vi "RemoveInterface.vi"(6 "InterfaceMethodsToRemove":string[](array[string])=["Add.Vi", "Execute.vi"], 7 "ClassWriter.lvclass":refnum<class "ClassWriter.lvclass">, 8 "error in":errorcluster, 9 "RemoveMethods":bool=TRUE, 10 "Interface Path":path=path "C:/Projects/Interface/Sub_Interface1/Sub_Interface1.lvclass", 11 "LvClassPath/LvClassProjectItem":variant) -> (0 "error out":errorcluster={"status"=TRUE, "code"=7, "source"="Invoke Node in InterfaceLibrary.lvlib:ImplementInterface.vi\n<APPEND>\nMethod Name: <b>LabVIEW Class:Open</b>"})   [LabVIEW 2020, in "InterfaceLibrary.lvlib"]
uses:
  InterfaceLibrary.lvlib
  Provider_BaseClassInterface/ClassWriter_class/ClassWriter.lvclass
  Provider_LvNativeClass/ClassWriterNative_class/ClassWriterNative.lvclass
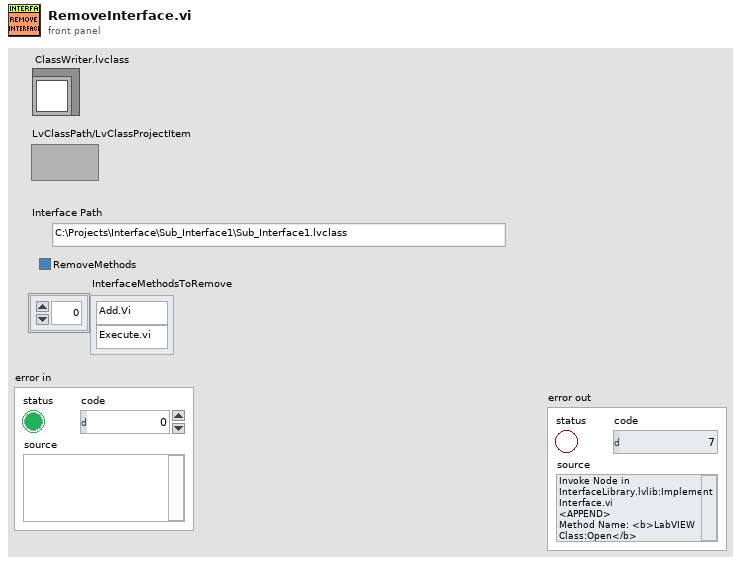
[diagram p1: front panel]
types:
  T1 = cluster{"ClassRef":refnum<vi>, "ClassRefCreated":bool, "Application":refnum<vi>, "InterfaceRef":refnum<vi>, "MethodsToImplement":path[], "MethodsDescription":string[], "MethodsScope":enum32{"invalid scope", "public", "private", "protected", "community"}[]}
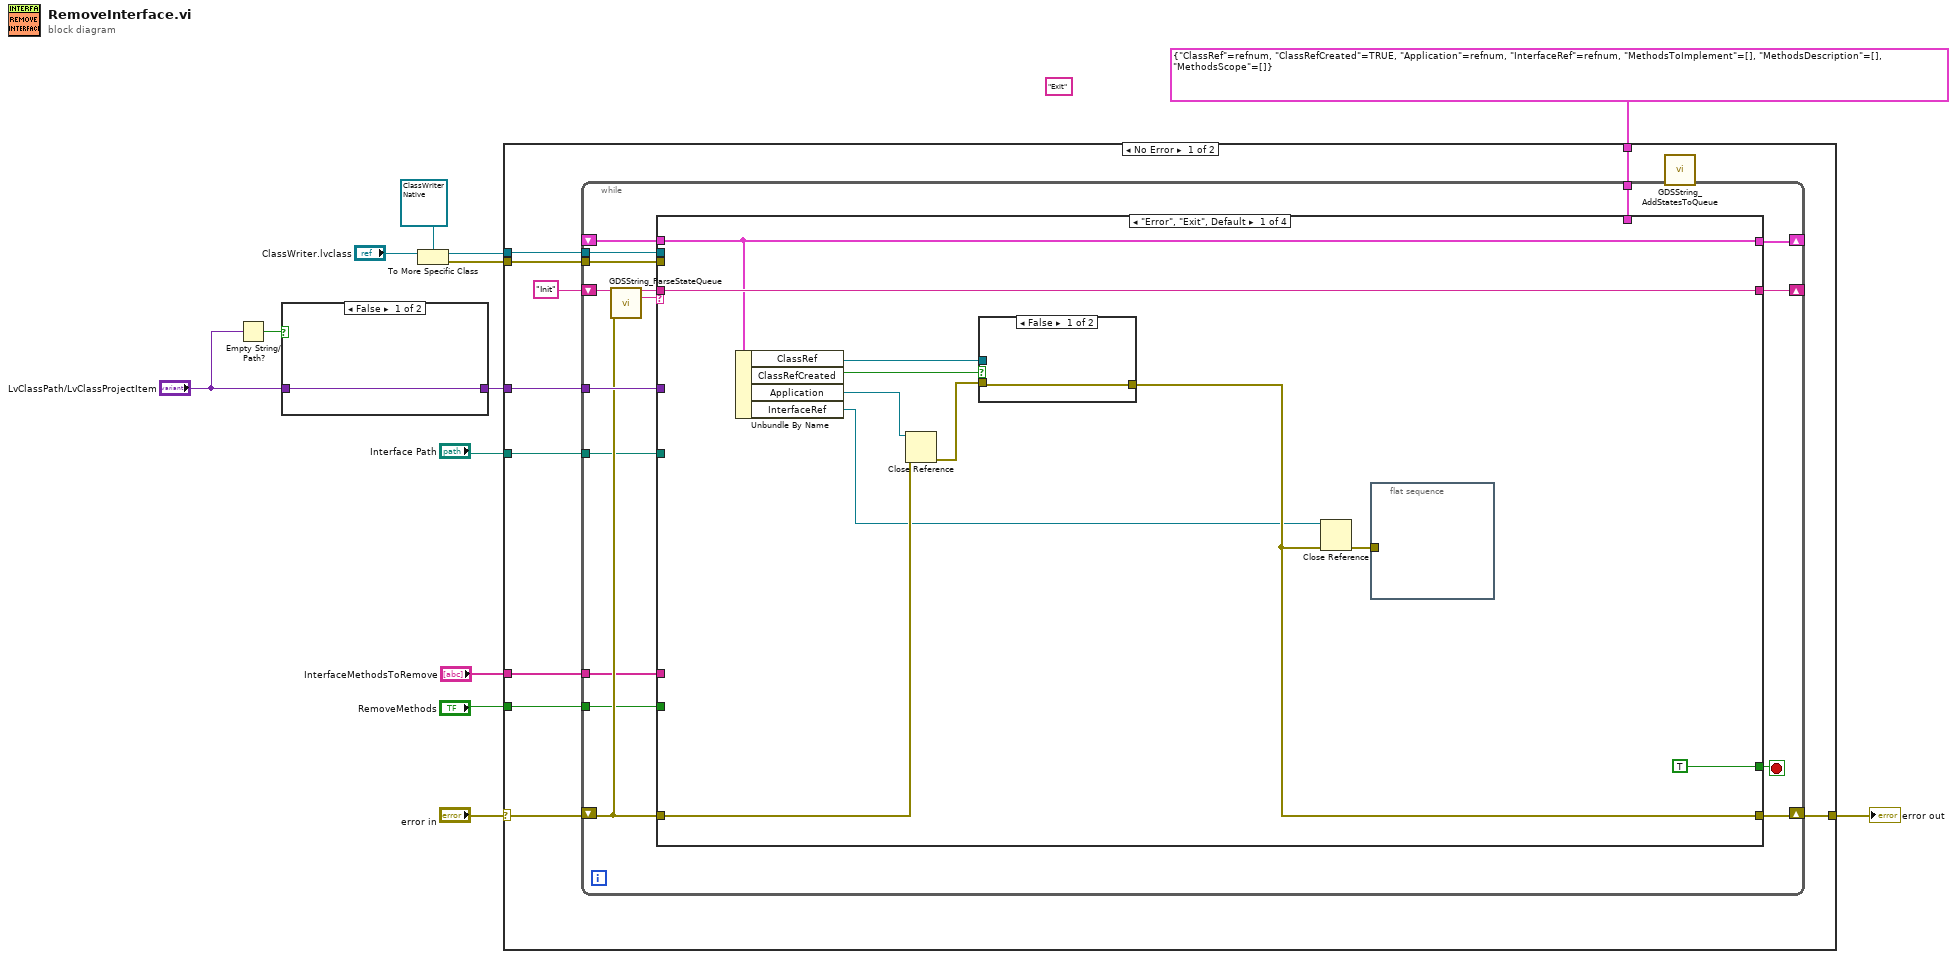
[diagram p0: block diagram]
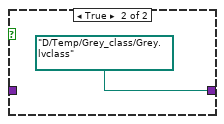
[diagram p2: hidden frame]
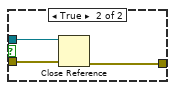
[diagram p3: hidden frame]
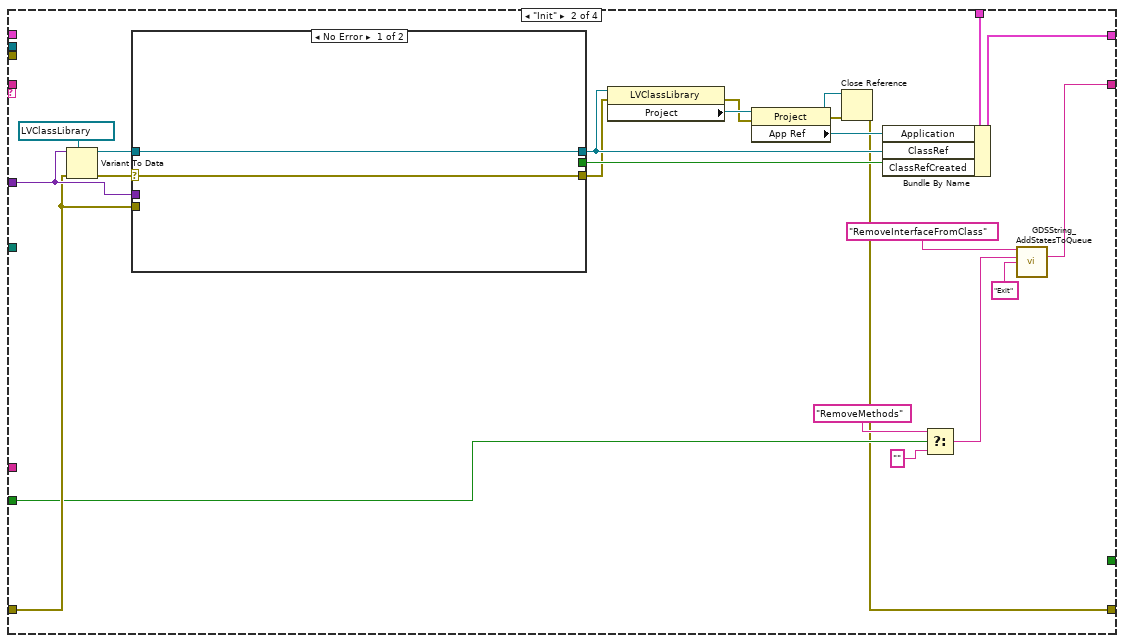
[diagram p4: hidden frame]
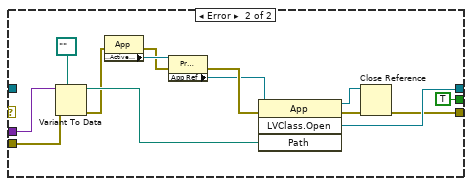
[diagram p5: hidden frame]
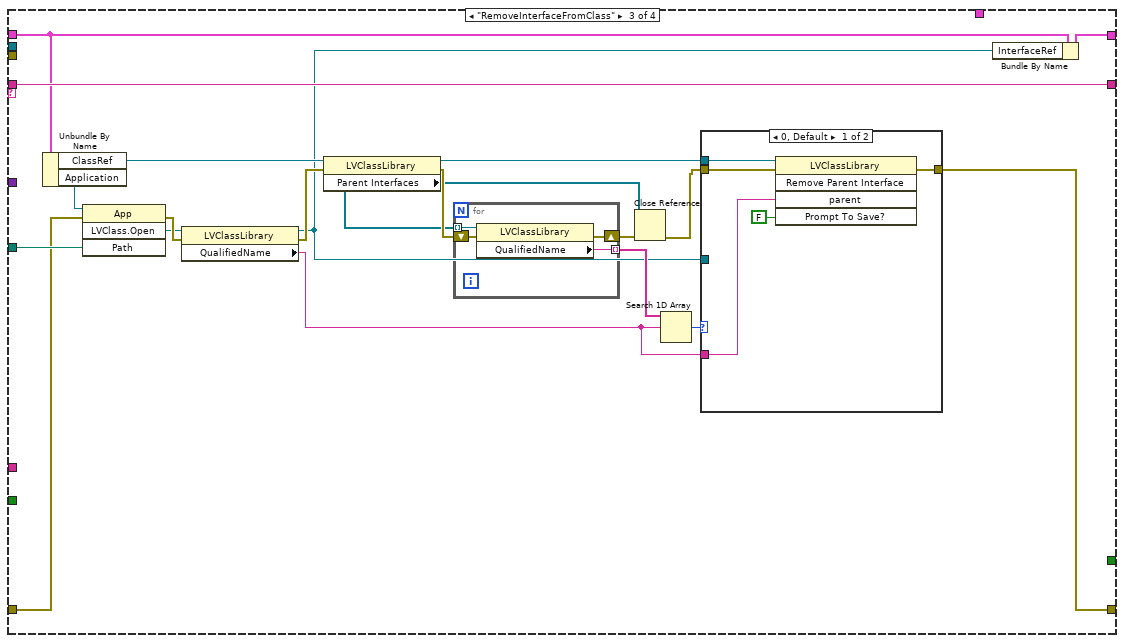
[diagram p6: hidden frame]
diagram:
  (unwired) "Exit" ("Remaining States")
  n1 = Empty String/Path?(string/path="LvClassPath/LvClassProjectItem") -> (empty?=w9:bool)
  n2 = case shown="False" w9 {
    tunnel: "LvClassPath/LvClassProjectItem" -> [w14 _]
    tunnel: [w14 path "D:/Temp/Grey_class/Grey.lvclass" ("Path")] -> w7
    frame False {
    }
    frame True {
    }
  }
  n3 = To More Specific Class(target class=refnum<class "ClassWriterNative.lvclass"> refnum ("ClassWriterNative"), reference="ClassWriter.lvclass") -> (specific class reference=w3:refnum<class "ClassWriterNative.lvclass">, error out=w1:errorcluster)  [unwired: 1 in]
  n4 = case shown="No Error" "error in" {
    selector: "error in" -> [w24 w128]
    tunnel: w7 -> [w25 _]
    tunnel: [w23 w128] -> w12
    tunnel: T1 {"ClassRef"=refnum, "ClassRefCreated"=TRUE, "Application"=refnum, "InterfaceRef"=refnum, "MethodsToImplement"=[], "MethodsDescription"=[], "MethodsScope"=[]} -> [w21 _]
    tunnel: "RemoveMethods" -> [w20 _]
    tunnel: "Interface Path" -> [w19 _]
    tunnel: "InterfaceMethodsToRemove" -> [w18 _]
    tunnel: w3 -> [w17 _]
    tunnel: w1 -> [w16 _]
    frame No Error {
      n5 = while {
        tunnel: w25 -> [w41]
        shift-right: [w40] -> w23
        shift-left: w24 -> [w38]
        shift-right: [w32] -> _
        shift-left: "Init" -> [w39]
        tunnel: w21 -> [w36]
        shift-right: [w35] -> _
        shift-left: _ -> [w34]
        tunnel: w20 -> [w30]
        tunnel: w19 -> [w29]
        tunnel: w18 -> [w28]
        tunnel: w17 -> [w27]
        tunnel: w16 -> [w26]
        stop <- w31 stop-if-true
        n6 = call "GDSString_ParseStateQueue.vi"("State Queue"=w39, "Error In (no error)"=w38) -> ("Remaining States"=w33:string, "Current State"=w37:string)  [unwired: 9 in, 3 out]
        n7 = case shown="\"Error\", \"Exit\", Default" w37 {
          tunnel: w41 -> [_ w76 _ _]
          tunnel: w38 -> [w45 w75 w107 w125]
          tunnel: [w44 w59 w108 w125] -> w40
          tunnel: [w50 w73 w106 w127] -> w35
          tunnel: w36 -> [_ w74 _ _]
          tunnel: w34 -> [w50 _ w113 w127]
          tunnel: [w52 w71 w114 w126] -> w32
          tunnel: w33 -> [w52 _ w114 w126]
          tunnel: [TRUE _ _ _] -> w31
          tunnel: w30 -> [_ w70 _ _]
          tunnel: w29 -> [_ _ w110 _]
          tunnel: w28 -> [_ _ _ _]
          tunnel: w27 -> [_ _ _ _]
          tunnel: w26 -> [_ _ _ _]
          frame "Error", "Exit", Default {
            n8 = Unbundle By Name(w50) -> ("ClassRef"=w48:refnum<vi>, "ClassRefCreated"=w49:bool, "Application"=w47:refnum<vi>, "InterfaceRef"=w43:refnum<vi>)
            n9 = Close Reference(reference=w47, error in (no error)=w45) -> (error out=w46:errorcluster)
            n10 = case shown="False" w49 {
              tunnel: w48 -> [_ w56]
              tunnel: w46 -> [w53 w55]
              tunnel: [w53 w54] -> w44
              frame False {
              }
              frame True {
                n11 = Close Reference(reference=w56, error in (no error)=w55) -> (error out=w54:errorcluster)
              }
            }
            n12 = Close Reference(reference=w43, error in (no error)=w44) -> (error out=w42:errorcluster)
            n13 = flat-sequence {
              tunnel: w42 -> [_]
              frame #0 {
              }
            }
          }
          frame "Init" {
            n14 = Variant To Data(error in=w75, type=refnum<vi> refnum ("ProjectItem"), Variant=w76) -> (data=w78:refnum<vi>, error out=w77:errorcluster)
            n15 = case shown="No Error" w77 {
              selector: w77 -> [w80 _]
              tunnel: w78 -> [w81 _]
              tunnel: [w80 w87] -> w60
              tunnel: w76 -> [_ w94]
              tunnel: w75 -> [_ w91]
              tunnel: [w81 w90] -> w64
              tunnel: [_ TRUE] -> w72
              frame No Error {
              }
              frame Error {
                n16 = Variant To Data(error in=w91, type=path "" ("Path"), Variant=w94) -> (data=w93:path, error out=w92:errorcluster)
                n17 = property class="App"(error in=w92) -> (error out=w84:errorcluster, "Project.ActiveProject"=w85:refnum<vi>)  [unwired: 1 in, 1 out]
                n18 = property class="Project"(reference=w85, error in=w84) -> (error out=w83:errorcluster, "App Ref"=w82:refnum<vi>)  [unwired: 1 out]
                n19 = invoke class="App" method="LVClass.Open"(reference=w82, error in=w83, "Path"=w93) -> (reference out=w88:refnum<vi>, error out=w89:errorcluster, "LVClass.Open"=w90:refnum<vi>)  [unwired: 1 in, 1 out]
                n20 = Close Reference(reference=w88, error in (no error)=w89) -> (error out=w87:errorcluster)
              }
            }
            n21 = property class="LVClassLibrary"(reference=w64, error in=w60) -> (error out=w57:errorcluster, "Project"=w58:refnum<vi>)  [unwired: 1 out]
            n22 = property class="Project"(reference=w58, error in=w57) -> (reference out=w62:refnum<vi>, error out=w61:errorcluster, "App Ref"=w63:refnum<vi>)
            n23 = Close Reference(reference=w62, error in (no error)=w61) -> (error out=w59:errorcluster)
            n24 = Bundle By Name(cluster=w74, "Application"=w63, "ClassRef"=w64, "ClassRefCreated"=w72) -> (w73:T1)
            n25 = Select(t="RemoveMethods" ("Remaining States"), s=w70, f="") -> (s? t:f=w66:string)
            n26 = call "GDSString_AddStatesToQueue.vi"("State(s) in Front (\"\")"="RemoveInterfaceFromClass" ("Remaining States"), "State(s) in (\"\")"=w66, "State(s) at Back (\"\")"="Exit" ("Remaining States")) -> ("States Out"=w71:string)  [unwired: 12 in]
          }
          frame "RemoveInterfaceFromClass" {
            n27 = Unbundle By Name(w113) -> ("ClassRef"=w112:refnum<vi>, "Application"=w111:refnum<vi>)
            n28 = invoke class="App" method="LVClass.Open"(reference=w111, error in=w107, "Path"=w110) -> (error out=w104:errorcluster, "LVClass.Open"=w101:refnum<vi>)  [unwired: 1 in, 2 out]
            n29 = property class="LVClassLibrary"(reference=w101, error in=w104) -> (error out=w103:errorcluster, "QualifiedName"=w96:string)  [unwired: 1 out]
            n30 = property class="LVClassLibrary"(reference=w112, error in=w103) -> (reference out=w109:refnum<vi>, error out=w99:errorcluster, "Parent Interfaces"=w97:refnum<vi>[])
            n31 = for {
              tunnel: w97 -> [w118] mode=indexing
              tunnel: [w117] -> w102 mode=indexing
              shift-right: [w116] -> w100
              shift-left: w99 -> [w115]
              n32 = property class="LVClassLibrary"(reference=w118, error in=w115) -> (error out=w116:errorcluster, "QualifiedName"=w117:string)  [unwired: 1 out]
            }
            n33 = Close Reference(reference=w97, error in (no error)=w100) -> (error out=w98:errorcluster)
            n34 = Search 1D Array(1D array=w102, element=w96) -> (index of element=w105:i32)  [unwired: 1 in]
            n35 = case shown="0, Default" w105 {
              tunnel: w109 -> [w123 _]
              tunnel: w98 -> [w119 w124]
              tunnel: w101 -> [_ _]
              tunnel: [w122 w124] -> w108
              tunnel: w96 -> [w120 _]
              frame 0, Default {
                n36 = invoke class="LVClassLibrary" method="Remove Parent Interface"(reference=w123, error in=w119, "parent"=w120, "Prompt To Save?"=FALSE) -> (error out=w122:errorcluster)  [unwired: 1 in, 4 out]
              }
              frame -1 {
              }
            }
            n37 = Bundle By Name(cluster=w113, "InterfaceRef"=w101) -> (w106:T1)
          }
          frame "RemoveMethods" {
          }
        }
      }
      n38 = call "GDSString_AddStatesToQueue.vi"() -> ()  [unwired: 15 in, 1 out]
    }
    frame Error {
    }
  }
  "error out" <- w12
